vi "create_column_names.vi"(1 "Pressure":enum16{"None", "Uncorrelated", "Correlated"}(ring), 2 "Velocity components":string, 3 "Concentration":enum16{"None", "Uncorrelated", "Correlated"}(ring)) -> (0 "Array":string[](array[string]))   [LabVIEW 2022 SP3]
panel:
  in  "Array 3":string[](array[string])
  in  "Array 2":string[](array[string])
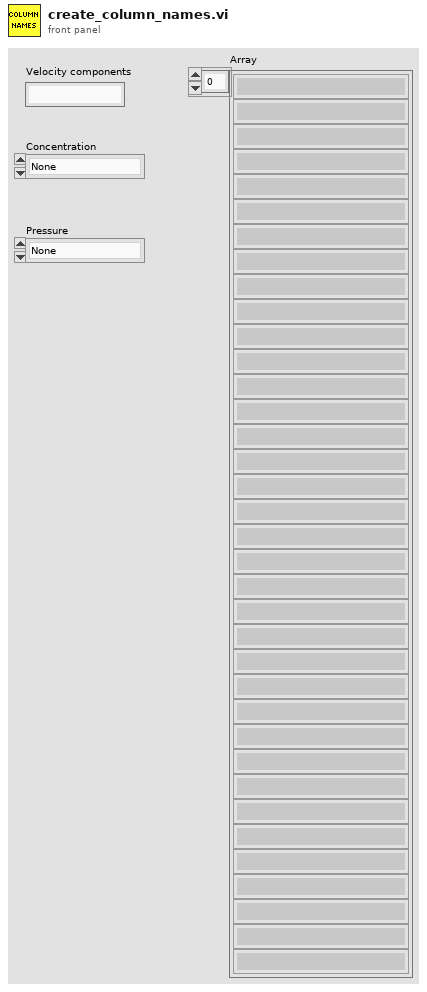
[diagram p1: front panel]
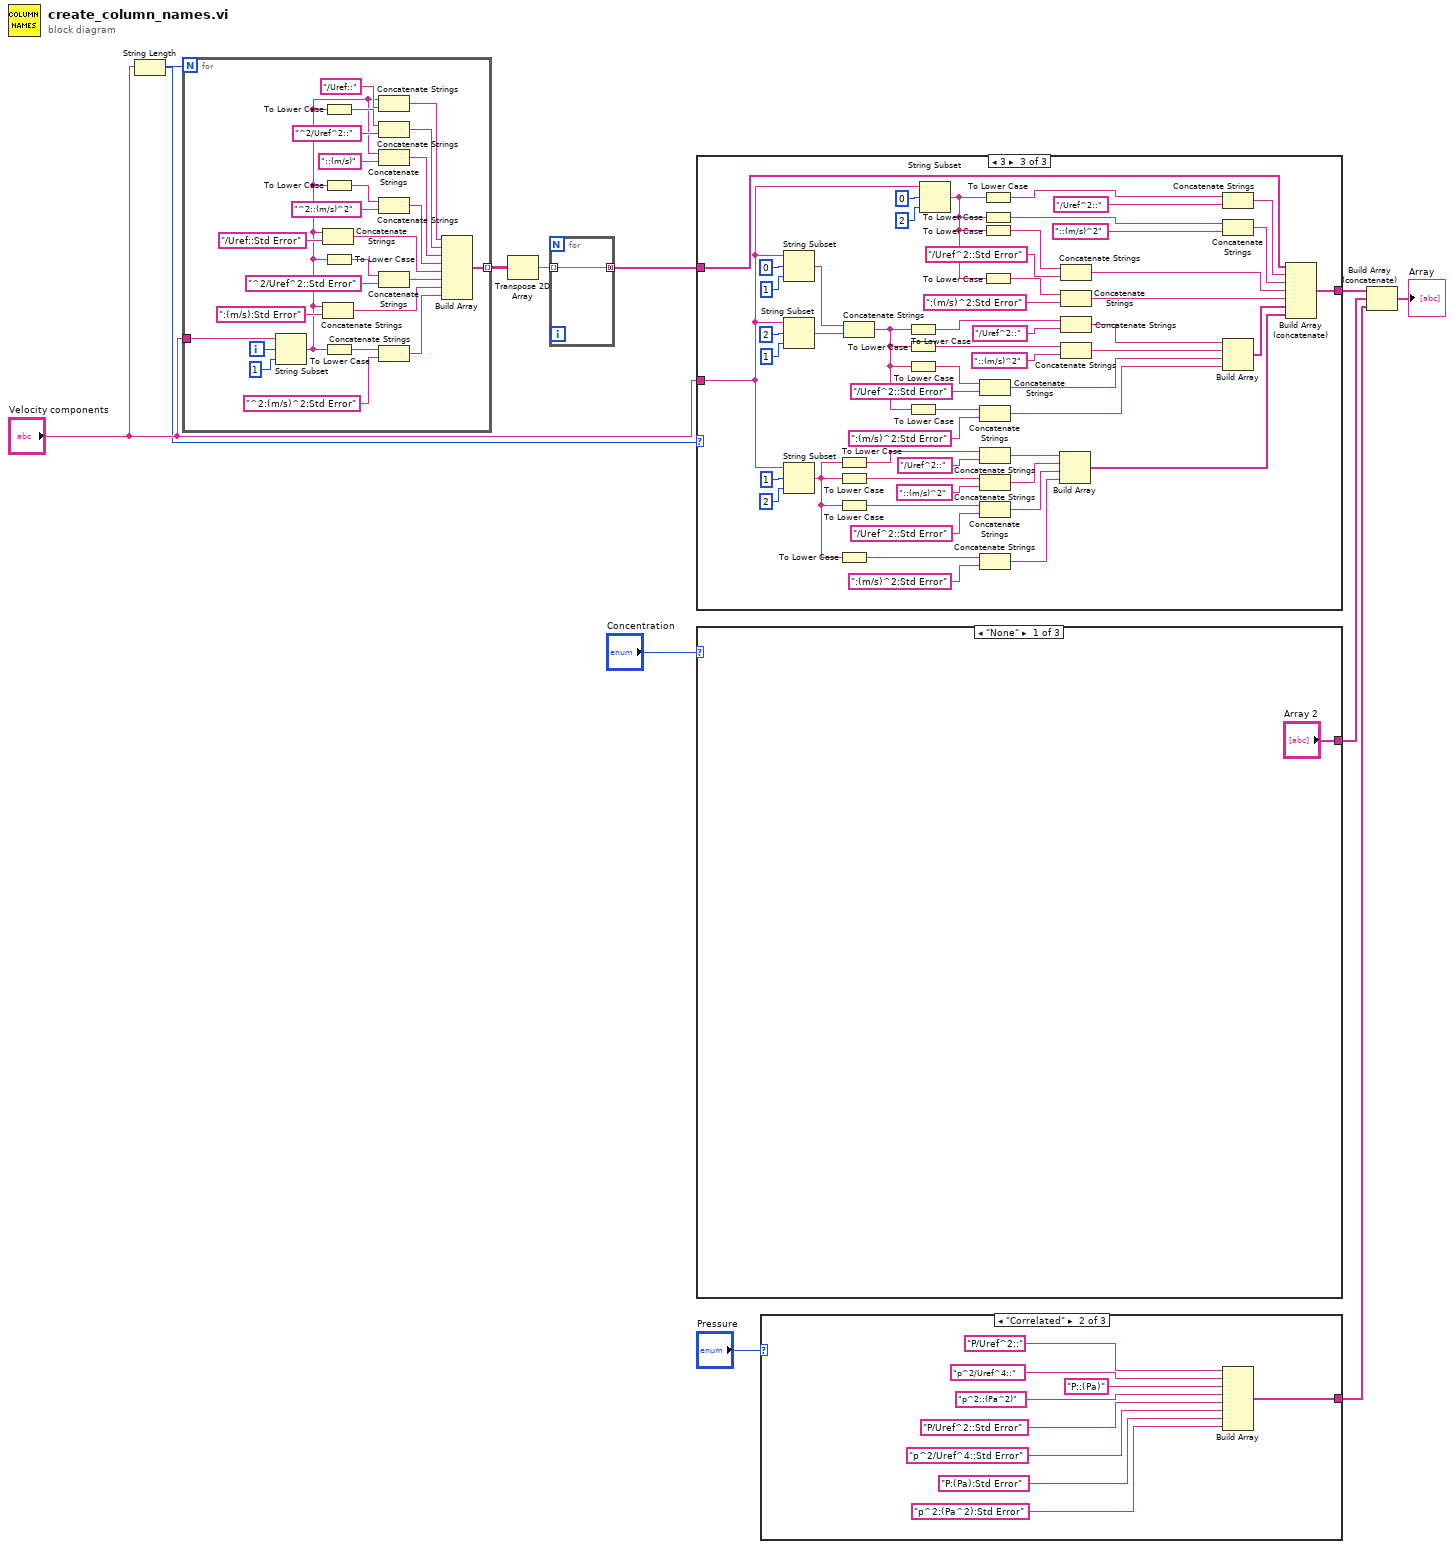
[diagram p0: block diagram]
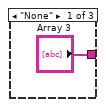
[diagram p2: hidden frame]
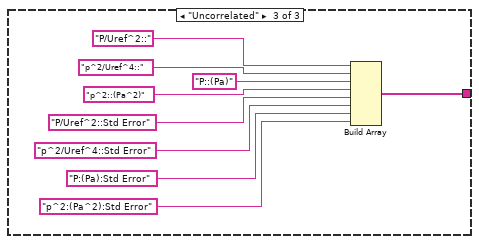
[diagram p3: hidden frame]
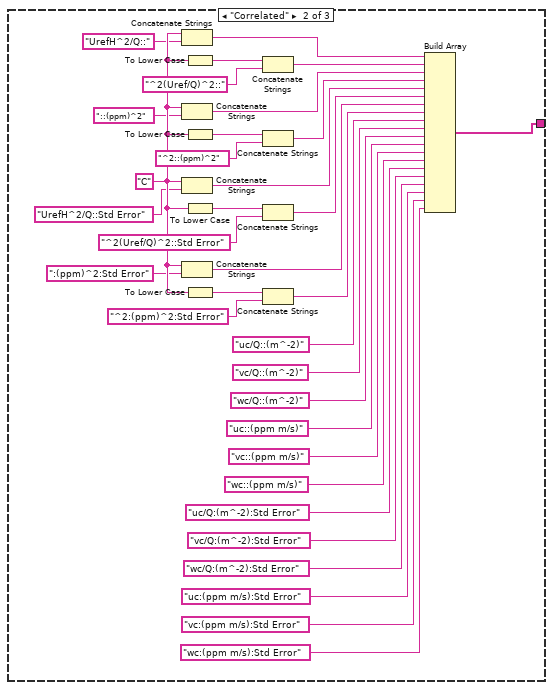
[diagram p4: hidden frame]
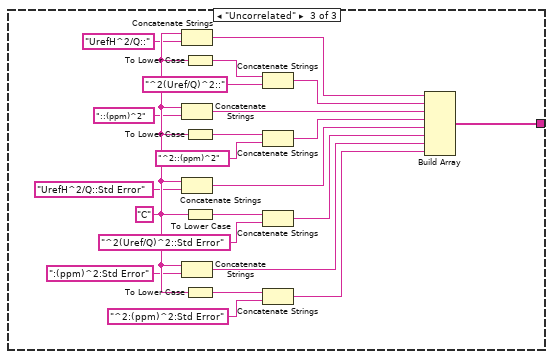
[diagram p5: hidden frame]
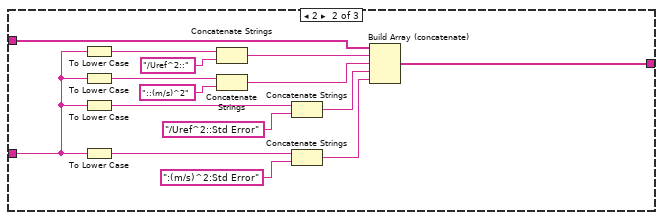
[diagram p7: hidden frame]
diagram:
  n1 = String Length(string="Velocity components") -> (length=w10:i32)
  n2 = for {
    N: w10 -> [_]
    tunnel: [w27] -> w9 mode=indexing
    tunnel: "Velocity components" -> [w22]
    i -> [w20]
    n3 = String Subset(string=w22, offset (0)=w20, length (rest)=1 ("length (rest)")) -> (substring=w23:string)
    n4 = Concatenate Strings(w23, "/Uref::Std Error" ("string")) -> (w15:string)
    n5 = Concatenate Strings(w23, ":(m/s):Std Error" ("string")) -> (w13:string)
    n6 = To Lower Case(string=w23) -> (all lower case string=w31:string)
    n7 = To Lower Case(string=w23) -> (all lower case string=w30:string)
    n8 = To Lower Case(string=w23) -> (all lower case string=w26:string)
    n9 = To Lower Case(string=w23) -> (all lower case string=w24:string)
    n10 = Concatenate Strings(w23, "/Uref::" ("string")) -> (w19:string)
    n11 = Concatenate Strings(w31, "^2/Uref^2::" ("string")) -> (w18:string)
    n12 = Concatenate Strings(w23, "::(m/s)" ("string")) -> (w17:string)
    n13 = Concatenate Strings(w30, "^2::(m/s)^2" ("string")) -> (w16:string)
    n14 = Concatenate Strings(w26, "^2/Uref^2::Std Error" ("string")) -> (w14:string)
    n15 = Concatenate Strings(w24, "^2:(m/s)^2:Std Error" ("string")) -> (w12:string)
    n16 = Build Array(w19, w18, w17, w16, w15, w14, w13, w12) -> (w27:string[])
  }
  n17 = Transpose 2D Array(2D array=w9) -> (transposed array=w7:string[][])
  n18 = for {
    tunnel: [w37] -> w8 mode=concatenating
    tunnel: w7 -> [w37] mode=indexing
  }
  n19 = case shown="3" w10 {
    tunnel: "Velocity components" -> [_ w45 w69]
    tunnel: w8 -> [w38 w40 w95]
    tunnel: [w38 w39 w94] -> w6
    frame 1, Default {
    }
    frame 2 {
      n20 = To Lower Case(string=w45) -> (all lower case string=w52:string)
      n21 = To Lower Case(string=w45) -> (all lower case string=w51:string)
      n22 = To Lower Case(string=w45) -> (all lower case string=w48:string)
      n23 = To Lower Case(string=w45) -> (all lower case string=w47:string)
      n24 = Concatenate Strings(w52, "/Uref^2::" ("string")) -> (w44:string)
      n25 = Concatenate Strings(w51, "::(m/s)^2" ("string")) -> (w43:string)
      n26 = Concatenate Strings(w48, "/Uref^2::Std Error" ("string")) -> (w42:string)
      n27 = Concatenate Strings(w47, ":(m/s)^2:Std Error" ("string")) -> (w41:string)
      n28 = Build Array (concatenate)(w40, w44, w43, w42, w41) -> (w39:string[])
    }
    frame 3 {
      n29 = String Subset(string=w69, offset (0)=0, length (rest)=1 ("length (rest)")) -> (substring=w71:string)
      n30 = String Subset(string=w69, offset (0)=2, length (rest)=1 ("length (rest)")) -> (substring=w70:string)
      n31 = String Subset(string=w69, offset (0)=1, length (rest)=2 ("length (rest)")) -> (substring=w76:string)
      n32 = To Lower Case(string=w76) -> (all lower case string=w83:string)
      n33 = To Lower Case(string=w76) -> (all lower case string=w84:string)
      n34 = To Lower Case(string=w76) -> (all lower case string=w87:string)
      n35 = To Lower Case(string=w76) -> (all lower case string=w88:string)
      n36 = Concatenate Strings(w71, w70) -> (w57:string)
      n37 = To Lower Case(string=w57) -> (all lower case string=w56:string)
      n38 = To Lower Case(string=w57) -> (all lower case string=w67:string)
      n39 = To Lower Case(string=w57) -> (all lower case string=w64:string)
      n40 = To Lower Case(string=w57) -> (all lower case string=w63:string)
      n41 = String Subset(string=w69, offset (0)=0, length (rest)=2 ("length (rest)")) -> (substring=w81:string)
      n42 = Concatenate Strings(w64, "/Uref^2::Std Error" ("string")) -> (w59:string)
      n43 = Concatenate Strings(w63, ":(m/s)^2:Std Error" ("string")) -> (w58:string)
      n44 = Concatenate Strings(w83, "/Uref^2::" ("string")) -> (w90:string)
      n45 = Concatenate Strings(w84, "::(m/s)^2" ("string")) -> (w91:string)
      n46 = Concatenate Strings(w87, "/Uref^2::Std Error" ("string")) -> (w92:string)
      n47 = Concatenate Strings(w88, ":(m/s)^2:Std Error" ("string")) -> (w93:string)
      n48 = To Lower Case(string=w81) -> (all lower case string=w106:string)
      n49 = To Lower Case(string=w81) -> (all lower case string=w105:string)
      n50 = To Lower Case(string=w81) -> (all lower case string=w102:string)
      n51 = To Lower Case(string=w81) -> (all lower case string=w101:string)
      n52 = Build Array(w90, w91, w92, w93) -> (w55:string[])
      n53 = Concatenate Strings(w102, "/Uref^2::Std Error" ("string")) -> (w97:string)
      n54 = Concatenate Strings(w101, ":(m/s)^2:Std Error" ("string")) -> (w96:string)
      n55 = Concatenate Strings(w56, "/Uref^2::" ("string")) -> (w61:string)
      n56 = Concatenate Strings(w67, "::(m/s)^2" ("string")) -> (w60:string)
      n57 = Concatenate Strings(w106, "/Uref^2::" ("string")) -> (w99:string)
      n58 = Concatenate Strings(w105, "::(m/s)^2" ("string")) -> (w98:string)
      n59 = Build Array(w61, w60, w59, w58) -> (w54:string[])
      n60 = Build Array (concatenate)(w95, w99, w98, w97, w96, w54, w55) -> (w94:string[])
    }
  }
  n61 = case shown="\"None\"" "Concentration" {
    tunnel: ["Array 2" w109 w143] -> w3
    frame "None" {
    }
    frame "Correlated" {
      w130 = "C"
      n62 = Concatenate Strings(w130, "UrefH^2/Q::" ("string")) -> (w133:string)
      n63 = Concatenate Strings(w130, "::(ppm)^2" ("string")) -> (w135:string)
      n64 = Concatenate Strings(w130, "UrefH^2/Q::Std Error" ("string")) -> (w137:string)
      n65 = Concatenate Strings(w130, ":(ppm)^2:Std Error" ("string")) -> (w140:string)
      n66 = To Lower Case(string=w130) -> (all lower case string=w131:string)
      n67 = To Lower Case(string=w130) -> (all lower case string=w132:string)
      n68 = To Lower Case(string=w130) -> (all lower case string=w138:string)
      n69 = To Lower Case(string=w130) -> (all lower case string=w141:string)
      n70 = Concatenate Strings(w131, "^2(Uref/Q)^2::" ("string")) -> (w134:string)
      n71 = Concatenate Strings(w132, "^2::(ppm)^2" ("string")) -> (w136:string)
      n72 = Concatenate Strings(w138, "^2(Uref/Q)^2::Std Error" ("string")) -> (w139:string)
      n73 = Concatenate Strings(w141, "^2:(ppm)^2:Std Error" ("string")) -> (w142:string)
      n74 = Build Array(w133, w134, w135, w136, w137, w139, w140, w142, "uc/Q::(m^-2)" ("string"), "vc/Q::(m^-2)" ("string"), "wc/Q::(m^-2)" ("string"), "uc::(ppm m/s)" ("string"), "vc::(ppm m/s)" ("string"), "wc::(ppm m/s)" ("string"), "uc/Q:(m^-2):Std Error" ("string"), "vc/Q:(m^-2):Std Error" ("string"), "wc/Q:(m^-2):Std Error" ("string"), "uc:(ppm m/s):Std Error" ("string"), "vc:(ppm m/s):Std Error" ("string"), "wc:(ppm m/s):Std Error" ("string")) -> (w109:string[])
    }
    frame "Uncorrelated" {
      w164 = "C"
      n75 = Concatenate Strings(w164, "UrefH^2/Q::" ("string")) -> (w150:string)
      n76 = Concatenate Strings(w164, "::(ppm)^2" ("string")) -> (w152:string)
      n77 = Concatenate Strings(w164, "UrefH^2/Q::Std Error" ("string")) -> (w155:string)
      n78 = Concatenate Strings(w164, ":(ppm)^2:Std Error" ("string")) -> (w160:string)
      n79 = To Lower Case(string=w164) -> (all lower case string=w146:string)
      n80 = To Lower Case(string=w164) -> (all lower case string=w148:string)
      n81 = To Lower Case(string=w164) -> (all lower case string=w156:string)
      n82 = To Lower Case(string=w164) -> (all lower case string=w162:string)
      n83 = Concatenate Strings(w146, "^2(Uref/Q)^2::" ("string")) -> (w151:string)
      n84 = Concatenate Strings(w148, "^2::(ppm)^2" ("string")) -> (w153:string)
      n85 = Concatenate Strings(w156, "^2(Uref/Q)^2::Std Error" ("string")) -> (w158:string)
      n86 = Concatenate Strings(w162, "^2:(ppm)^2:Std Error" ("string")) -> (w163:string)
      n87 = Build Array(w150, w151, w152, w153, w155, w158, w160, w163) -> (w143:string[])
    }
  }
  n88 = case shown="\"Correlated\"" "Pressure" {
    tunnel: ["Array 3" w166 w183] -> w1
    frame "None" {
    }
    frame "Correlated" {
      n89 = Build Array("P/Uref^2::" ("string"), "p^2/Uref^4::" ("string"), "P::(Pa)" ("string"), "p^2::(Pa^2)" ("string"), "P/Uref^2::Std Error" ("string"), "p^2/Uref^4::Std Error" ("string"), "P:(Pa):Std Error" ("string"), "p^2:(Pa^2):Std Error" ("string")) -> (w166:string[])
    }
    frame "Uncorrelated" {
      n90 = Build Array("P/Uref^2::" ("string"), "p^2/Uref^4::" ("string"), "P::(Pa)" ("string"), "p^2::(Pa^2)" ("string"), "P/Uref^2::Std Error" ("string"), "p^2/Uref^4::Std Error" ("string"), "P:(Pa):Std Error" ("string"), "p^2:(Pa^2):Std Error" ("string")) -> (w183:string[])
    }
  }
  n91 = Build Array (concatenate)(w6, w3, w1) -> (→"Array":string[])
